vi "Acquire.vi"(6 "UI":refnum<queue>, 8 "error in (no error)":errorcluster, 9 "Data Queue 2":refnum<queue>, 10 "Data Notifier":refnum<notifier>, 11 "Hardware Resources in":T1={"VISA Refnum in"="", "Serial Configuration"={"Baud Rate"=460800, "Flow Control"=0}, "Voltage Level (0V)"=0.0, "Output Phase(s) (1-Phase)"=0, "Active Phase (1:Phase 1)"=1} {"Output Phase(s) (1-Phase)" items=["3 phase", "1 phase"]; "Active Phase (1:Phase 1)" items=["Phase 1"=1, "Phase 2"=2, "Phase 3"=3]; "Serial Configuration"."Flow Control" items=["None", "XON/XOFF", "RTS/CTS", "XON/XOFF & RTS/CTS", "DTR/DSR", "XON/XOFF & DTR/DSR"]; "Serial Configuration"."Baud Rate" items=["9600"=9600, "19200"=19200, "38400"=38400, "57600"=57600, "115200"=115200, "230400"=230400, "460800"=460800]}) -> (0 "error out":errorcluster, 3 "Hardware Resources out":T1={"VISA Refnum in"="", "Serial Configuration"={"Baud Rate"=460800, "Flow Control"=0}, "Voltage Level (0V)"=0.0, "Output Phase(s) (1-Phase)"=0, "Active Phase (1:Phase 1)"=1} {"Output Phase(s) (1-Phase)" items=["3 phase", "1 phase"]; "Active Phase (1:Phase 1)" items=["Phase 1"=1, "Phase 2"=2, "Phase 3"=3]; "Serial Configuration"."Flow Control" items=["None", "XON/XOFF", "RTS/CTS", "XON/XOFF & RTS/CTS", "DTR/DSR", "XON/XOFF & DTR/DSR"]; "Serial Configuration"."Baud Rate" items=["9600"=9600, "19200"=19200, "38400"=38400, "57600"=57600, "115200"=115200, "230400"=230400, "460800"=460800]})   [LabVIEW 2013, in "Cal Inst Acquisition.lvlib"]
doc: "Perform the acquisition. Replace the contents of this diagram with calls to acquisition hardware."
uses:
  Cal Inst Acquisition.lvlib
  Hardware Configuration.ctl
  controls/electrical2.ctl
  support/Message Queue/Message Cluster.ctl
  support/Message Queue/Cal Inst Message Queue.lvlib
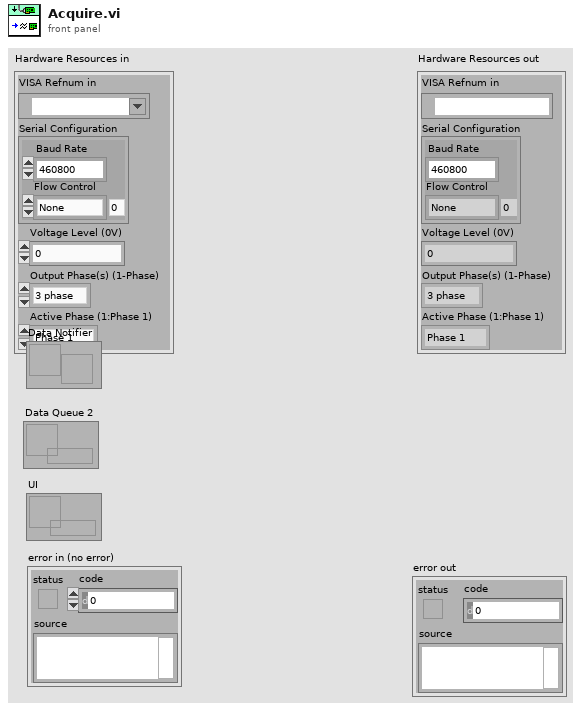
[diagram p1: front panel]
types:
  T1 = typedef "Cal Inst Acquisition.lvlib/Hardware Configuration.ctl" = cluster{"VISA Refnum in":refnum<visa-resource-name>, "Serial Configuration":cluster{"Baud Rate":u32, "Flow Control":u16}, "Voltage Level (0V)":dbl, "Output Phase(s) (1-Phase)":u16, "Active Phase (1:Phase 1)":i32}
  T2 = typedef "Cal Inst Acquisition.lvlib/electrical2.ctl" = cluster{"Time Stamp":timestamp, "Temperature (C)":dbl, "Electrical Data":string[][], "Waveform Graph":waveform(dbl)[]}
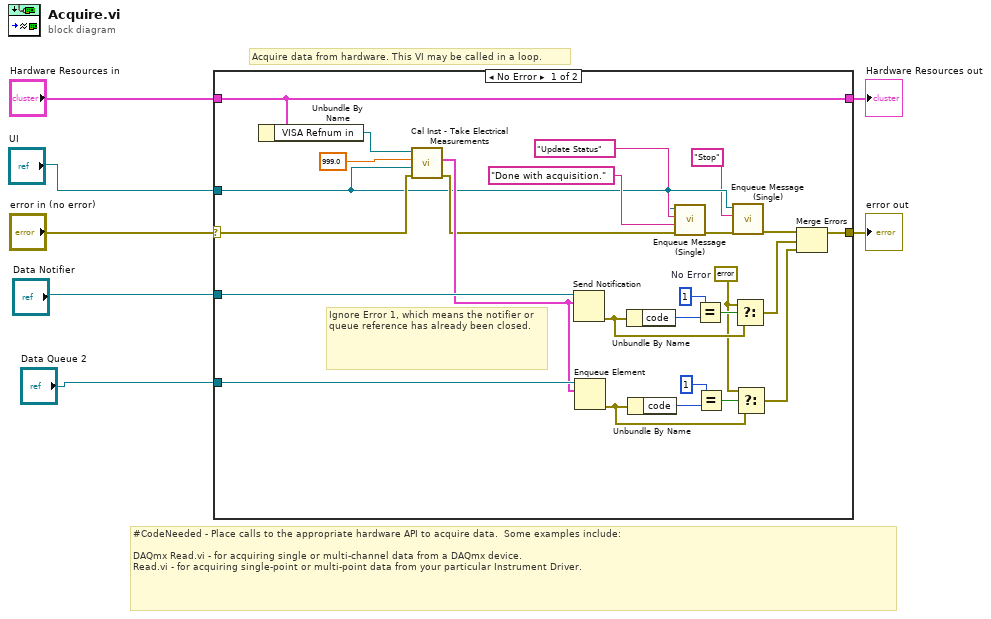
[diagram p0: block diagram]
diagram:
  # "Acquire data from hardware. This VI may be called in a loop."
  # "#CodeNeeded - Place calls to the appropriate hardware API to acquire data.  Some examples include:\n\nDAQmx Read.vi - for acquiring single or multi-channel data from a DAQmx device.\nRead.vi - for acquiring single-point or multi-point data from your particular Instrument Driver."
  n1 = case shown="No Error" "error in (no error)" {
    selector: "error in (no error)" -> [w16 w34]
    tunnel: [w33 w34] -> w6
    tunnel: "Hardware Resources in" -> [w19 w35]
    tunnel: [w19 w35] -> w4
    tunnel: "Data Notifier" -> [w32 _]
    tunnel: "Data Queue 2" -> [w21 _]
    tunnel: "UI" -> [w9 _]
    frame No Error {
      w20 = errorcluster {"status"=FALSE, "code"=0, "source"=""}  # No Error
      # "Ignore Error 1, which means the notifier or queue reference has already been closed."
      n2 = Unbundle By Name(w19) -> ("VISA Refnum in"=w18:refnum<visa-resource-name>)
      n3 = call "Cal Inst - Take Electrical Measurements.vi"("error in (no error)"=w16, "UI"=w9, "Temperature in"=999.0, "VISA Refnum in"=w18) -> ("error out"=w14:errorcluster, "Electrical Data 2"=w17:T2)  [unwired: 5 in, 1 out]
      n4 = Send Notification(notification=w17, notifier=w32) -> (error out=w28:errorcluster)  [unwired: 1 in, 1 out]
      n5 = Enqueue Element(queue=w21, element=w17) -> (error out=w26:errorcluster)  [unwired: 2 in, 2 out]
      n6 = Unbundle By Name(w28) -> ("code"=w31:i32)
      n7 = Unbundle By Name(w26) -> ("code"=w23:i32)
      n8 = call "Enqueue Message (Single).vi"("error in (no error)"=w14, "Message Data"="Done with acquisition." ("Message"), "Message"="Update Status", "Message Queue"=w9) -> ("error out"=w11:errorcluster)  [unwired: 6 in, 1 out]
      n9 = Equal?(x=1, y=w31) -> (x = y?=w29:bool)
      n10 = Equal?(x=1, y=w23) -> (x = y?=w25:bool)
      n11 = call "Enqueue Message (Single).vi"("error in (no error)"=w11, "Message"="Stop", "Message Queue"=w9) -> ("error out"=w10:errorcluster)  [unwired: 7 in, 1 out]
      n12 = Select(t=w20, s=w29, f=w28) -> (s? t:f=w27:errorcluster)
      n13 = Select(t=w20, s=w25, f=w26) -> (s? t:f=w22:errorcluster)
      n14 = Merge Errors(w10, w27, w22) -> (w33:errorcluster)
    }
    frame Error {
    }
  }
  "Hardware Resources out" <- w4
  "error out" <- w6
